vi "timer.vi"(8 "error in":errorcluster, 10 "limit":dbl, 11 "timer status":T1) -> (0 "error out":errorcluster, 2 "time":dbl, 3 "elapsed":bool)   [LabVIEW 2015]
uses:
  Controls/timer status.ctl
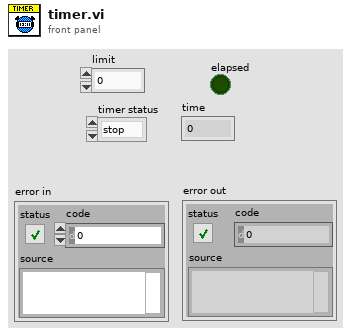
[diagram p1: front panel]
types:
  T1 = typedef "timer status.ctl" = enum16{"stop", "start"}
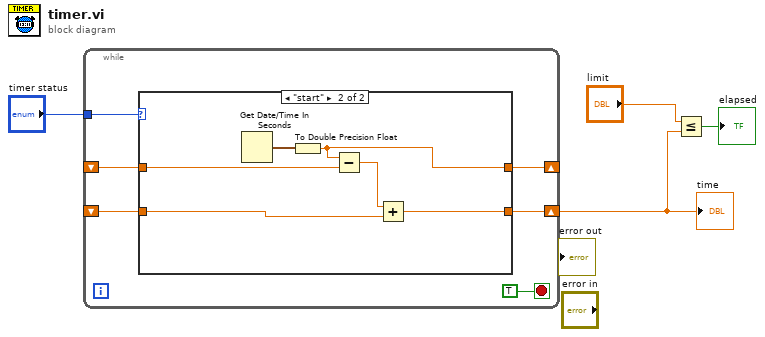
[diagram p0: block diagram]
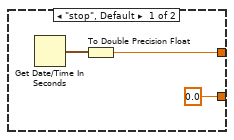
[diagram p2: hidden frame]
diagram:
  n1 = while {
    tunnel: "timer status" -> [w10]
    shift-right: [w9] -> _
    shift-left: _ -> [w6]
    shift-right: [w7] -> w2
    shift-left: _ -> [w5]
    stop <- TRUE stop-if-true
    n2 = case shown="\"start\"" w10 {
      tunnel: [w12 w14] -> w9
      tunnel: [0.0 w15] -> w7
      tunnel: w6 -> [_ w18]
      tunnel: w5 -> [_ w16]
      frame "stop", Default {
        n3 = Get Date/Time In Seconds() -> (seconds since 1Jan1904=w13:timestamp)
        n4 = To Double Precision Float(number=w13) -> (double precision float=w12:dbl)
      }
      frame "start" {
        n5 = Get Date/Time In Seconds() -> (seconds since 1Jan1904=w19:timestamp)
        n6 = To Double Precision Float(number=w19) -> (double precision float=w14:dbl)
        n7 = Subtract(x=w14, y=w18) -> (x-y=w17:dbl)
        n8 = Add(x=w17, y=w16) -> (x+y=w15:dbl)
      }
    }
  }
  "time" <- w2
  n9 = Less Or Equal?(x="limit", y=w2) -> (x <= y?=→"elapsed":bool)
